vi "Insert_data.vi"(8 "input data":variant, 10 "table":string, 11 "columns":string[](array[string])) -> (0 "connection reference out":T1, 1 "Application Directory":path, 2 "connection information":path, 3 "error out":errorcluster)   [LabVIEW 2014]
doc: "Block is used to insert row to databse table"
uses:
  <vilib>/addons/database/Connection.llb/Conn ObjectReference.ctl
  <vilib>/addons/database/Connection.llb/DB Tools Open Connec (Path).vi
  <vilib>/addons/database/NI_Database_API.lvlib
panel:
  # "Block is used to insert row to databse table"
  # "Outputs"
  # "Inputs"
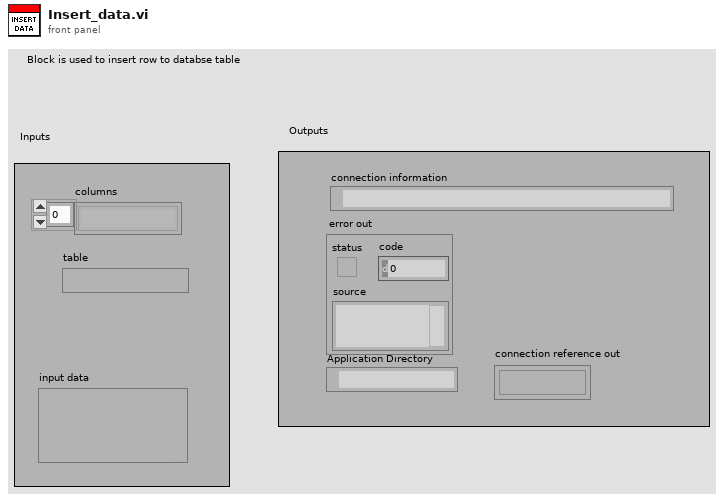
[diagram p1: front panel]
types:
  T1 = typedef "NI_Database_API.lvlib/Conn ObjectReference.ctl" = refnum<k1>
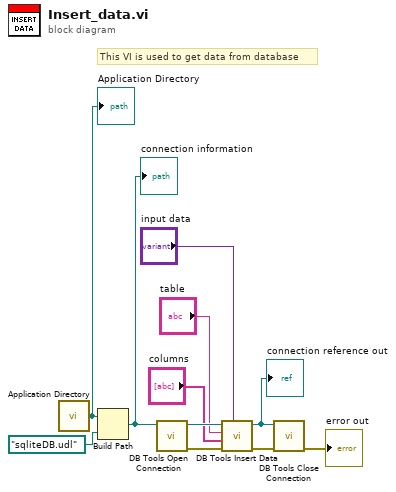
[diagram p0: block diagram]
diagram:
  # "This VI is used to get data from database"
  n1 = call <vilib>:"Application Directory.vi"() -> ("Application Directory"=w9:path)
  "Application Directory" <- w9
  n2 = Build Path(base path=w9, name or relative path=path "sqliteDB.udl" ("connection information")) -> (appended path=w8:path)
  "connection information" <- w8
  n3 = call-poly <vilib>:"DB Tools Open Connection.vi"("connection information"=w8) -> ("error out"=w10:errorcluster, "connection reference"=w11:T1)  [unwired: 7 in]
  n4 = call <vilib>:"DB Tools Insert Data.vi"("data"="input data", "error in (no error)"=w10, "columns"="columns", "table"="table", "connection reference"=w11) -> ("error out"=w3:errorcluster, "connection reference out"=w4:T1)  [unwired: 5 in]
  "connection reference out" <- w4
  n5 = call <vilib>:"DB Tools Close Connection.vi"("error in (no error)"=w3, "connection reference"=w4) -> ("error out"=→"error out":errorcluster)  [unwired: 5 in]
